vi "TW Generate proto file.vi"(8 "error in":errorcluster, 10 "New Subname":string, 11 "Template Project Path":path) -> (0 "error out":errorcluster, 2 "gRPC Service Name":string, 3 "proto File Path":path)   [LabVIEW 2021, in "Plugin Generator.lvlib"]
uses:
  Plugin Generator.lvlib
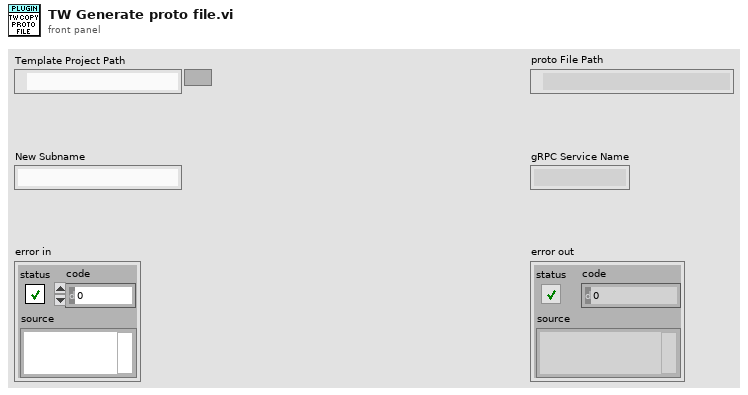
[diagram p1: front panel]
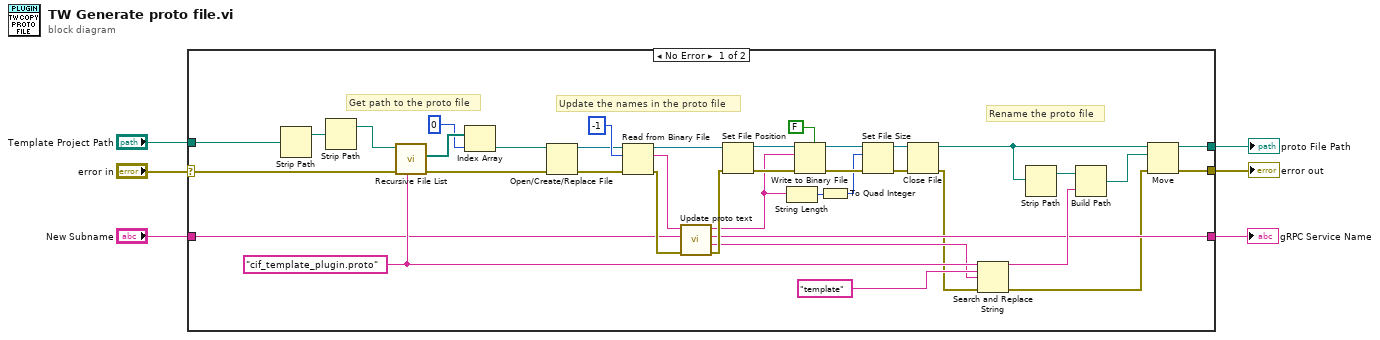
[diagram p0: block diagram]
diagram:
  n1 = case shown="No Error" "error in" {
    selector: "error in" -> [w23 w45]
    tunnel: [w30 w45] -> w6
    tunnel: [w29 _] -> w5
    tunnel: "New Subname" -> [w18 _]
    tunnel: "Template Project Path" -> [w22 _]
    tunnel: [w17 _] -> w1
    frame No Error {
      w41 = "cif_template_plugin.proto" ("pattern")
      # "Rename the proto file"
      # "Update the names in the proto file"
      # "Get path to the proto file"
      n2 = Strip Path(path=w22) -> (stripped path=w38:path)  [unwired: 1 out]
      n3 = Strip Path(path=w38) -> (stripped path=w37:path)  [unwired: 1 out]
      n4 = call <vilib>:"Recursive File List.vi"("pattern"=w41, "error in (no error)"=w23, "Folder Path"=w37) -> ("error out"=w28:errorcluster, "All Files in Dir"=w44:path[])  [unwired: 4 in, 3 out]
      n5 = Index Array(array=w44, index=0) -> (element=w24:path)
      n6 = Open/Create/Replace File(file path (use dialog)=w24, error in=w28) -> (refnum out=w25:refnum<file>, error out=w27:errorcluster)  [unwired: 4 in, 1 out]
      n7 = Read from Binary File(8:w27, 10:-1 ("count (1)"), 11:w25) -> (0:w19:errorcluster, 2:w21:string, 3:w35:refnum<file>)  [unwired: 3 in, 1 out]
      n8 = call "Update proto text.vi"("error in"=w19, "New Subname"=w18, "Proto Text In"=w21) -> ("error out"=w20:errorcluster, "snake_case"=w16:string, "gRPC Service Name"=w17:string, "Proto Text Out"=w9:string)  [unwired: 5 in]
      n9 = Set File Position(refnum=w35, error in=w20) -> (refnum out=w34:refnum<file>, error out=w33:errorcluster)  [unwired: 2 in]
      n10 = String Length(string=w9) -> (length=w8:i32)
      n11 = Write to Binary File(file (use dialog)=w34, data=w9, error in=w33, 5:FALSE ("prepend array or string size? (T)")) -> (refnum out=w13:refnum<file>, error out=w12:errorcluster)  [unwired: 2 in, 1 out]
      n12 = To Quad Integer(1:w8) -> (0:w7:i64)
      n13 = Set File Size(4:w12, 6:w7, 7:w13) -> (0:w11:errorcluster, 3:w10:refnum<file>)
      n14 = Close File(refnum=w10, error in=w11) -> (path=w32:path, error out=w15:errorcluster)
      n15 = Search and Replace String(input string=w41, search string="template", replace string=w16, error in=w15) -> (result string=w39:string, error out=w14:errorcluster)  [unwired: 4 in, 2 out]
      n16 = Strip Path(path=w32) -> (stripped path=w36:path)  [unwired: 1 out]
      n17 = Build Path(base path=w36, name or relative path=w39) -> (appended path=w31:path)
      n18 = Move(source path=w32, error in=w14, 10:w31) -> (error out=w30:errorcluster, 3:w29:path)  [unwired: 2 in, 1 out]
    }
    frame Error {
    }
  }
  "error out" <- w6
  "proto File Path" <- w5
  "gRPC Service Name" <- w1
